vi "GetClassTemplates.vi"(0 "ClassWriterNative in":refnum<class "ClassWriterNative.lvclass">, 1 "DerivedFromThisClass(if any)":refnum<vi>, 5 "error in (no error)":errorcluster) -> (14 "ClassWriterNative out":refnum<class "ClassWriterNative.lvclass">, 15 "Templates":T1[](array[typedef]), 19 "error out":errorcluster)   [LabVIEW 2014, in "ClassWriterNative.lvclass"]
uses:
  <resource>/Framework/Providers/Open_GDS/ClassProviders/Provider_LvNativeClass/ClassWriterNative_class/ClassWriterNative.lvclass
  <resource>/Framework/Providers/Open_GDS/ClassProviders/Provider_BaseClassInterface/ClassTemplateType.ctl
  <resource>/Framework/Providers/Open_GDS/ClassProviders/Common/ScriptingFunctions/Scripting_ConnectorPanePatternType.ctl
  <resource>/Framework/Providers/Open_GDS/ClassProviders/Provider_BaseClassInterface/ClassWriter_class/ClassWriter.lvclass
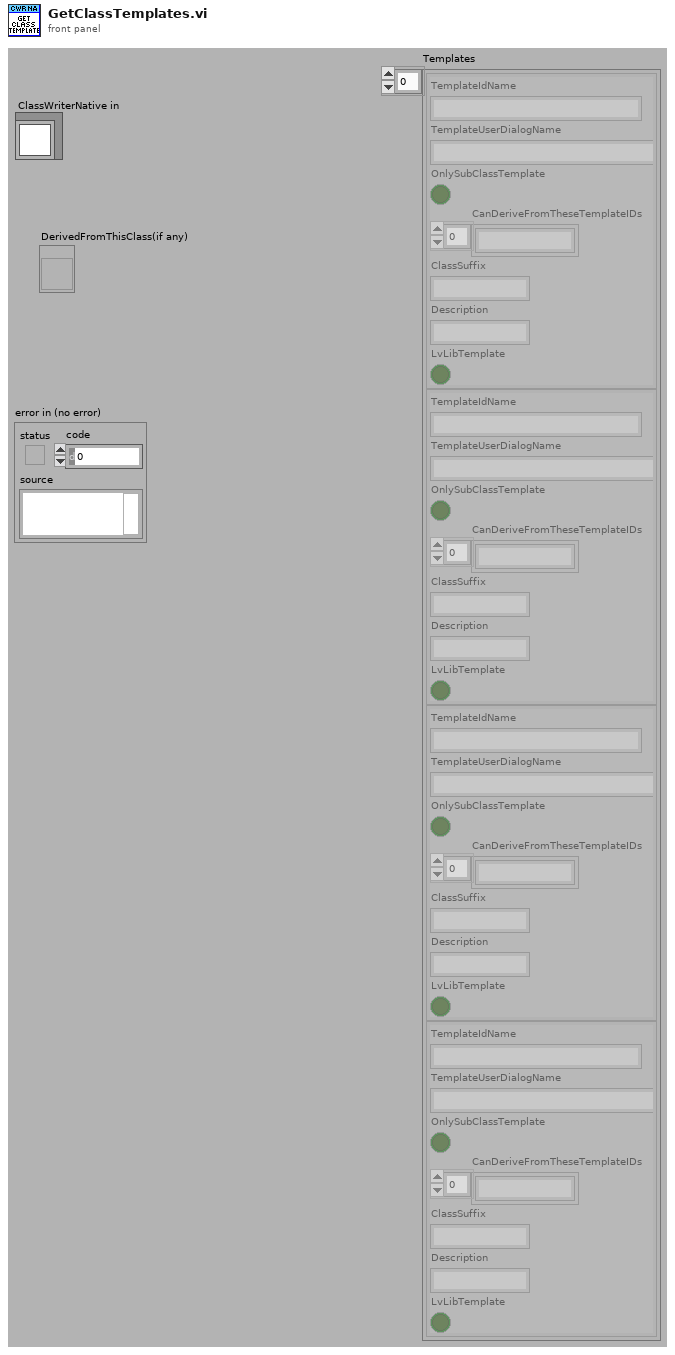
[diagram p1: front panel]
types:
  T1 = typedef "ClassWriter.lvclass/ClassTemplateType.ctl" = cluster{"TemplateIdName":string, "TemplateUserDialogName":string, "OnlySubClassTemplate":bool, "CanDeriveFromTheseTemplateIDs":string[], "ClassSuffix":string, "Description":string, "LvLibTemplate":bool}
  T2 = typedef "Scripting_ConnectorPanePatternType.ctl" = u16
  T3 = typedef "GDSLvCLass_ClassSettingsType.ctl" = cluster{"ClassProviderName":string, "ClassTemplateUsed":string, "ClassTemplateVersion":string, "ClassDescription":string, "PlugIns":T4[], "ConnectorPanePattern":string}
  T4 = typedef "GDSLvClass_PlugIn.ctl" = cluster{"Type":T5, "ID":string, "Version":string, "Path":path, "Name":string, "Data":variant}
  T5 = typedef "GDSLvClass_PlugInTypes.ctl" = enum16{"DesignPattern", "MethodTypes"}
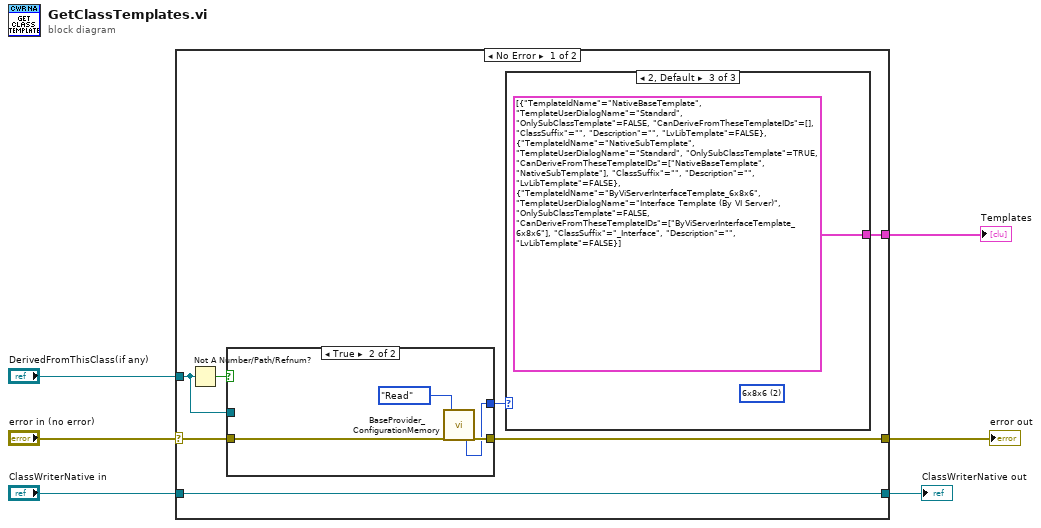
[diagram p0: block diagram]
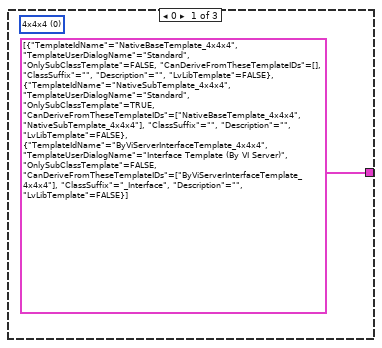
[diagram p2: hidden frame]
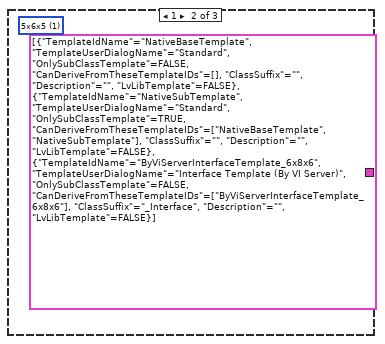
[diagram p3: hidden frame]
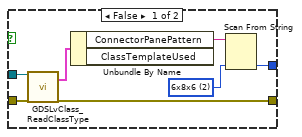
[diagram p4: hidden frame]
diagram:
  n1 = case shown="No Error" "error in (no error)" {
    selector: "error in (no error)" -> [w9 w29]
    tunnel: [w8 w29] -> w5
    tunnel: [w13 w28] -> w3
    tunnel: "ClassWriterNative in" -> [w13 w28]
    tunnel: [w12 _] -> w2
    tunnel: "DerivedFromThisClass(if any)" -> [w10 _]
    frame No Error {
      n2 = Not A Number/Path/Refnum?(number/path/refnum=w10) -> (NaN/Path/Refnum?=w11:bool)
      n3 = case shown="True" w11 {
        tunnel: w9 -> [w20 w26]
        tunnel: w10 -> [w19 _]
        tunnel: [w18 w25] -> w8
        tunnel: [w17 w24] -> w7
        frame False {
          w21 = T2 2 items=["4x4x4", "5x6x5", "6x8x6"] ("Pattern")
          n4 = call <resource>:"GDSLvClass_ReadClassType.vi"("Class Refnum In"=w19, "error in (no error)"=w20) -> ("ClassSettings"=w23:T3, "error out"=w18:errorcluster)  [unwired: 15 in, 1 out]
          n5 = Unbundle By Name(w23) -> ("ConnectorPanePattern"=w22:string)  [unwired: 1 out]
          n6 = Scan From String(input string=w22, default 1=w21) -> (output 1=w17:T2)  [unwired: 3 in, 3 out]
        }
        frame True {
          n7 = call <resource>:"BaseProvider_ConfigurationMemory.vi"("error in (no error)"=w26, "Action"=enum16{"Read", "Load", "Save"}."Read") -> ("PatternOut"=w24:T2, "error out"=w25:errorcluster)  [unwired: 11 in, 5 out]
        }
      }
      n8 = case shown="2, Default" w7 {
        tunnel: [T1[] [{"TemplateIdName"="NativeBaseTemplate_4x4x4", "TemplateUserDialogName"="Standard", "OnlySubClassTemplate"=FALSE, "CanDeriveFromTheseTemplateIDs"=[], "ClassSuffix"="", "Description"="", "LvLibTemplate"=FALSE}, {"TemplateIdName"="NativeSubTemplate_4x4x4", "TemplateUserDialogName"="Standard", "OnlySubClassTemplate"=TRUE, "CanDeriveFromTheseTemplateIDs"=["NativeBaseTemplate_4x4x4", "NativeSubTemplate_4x4x4"], "ClassSuffix"="", "Description"="", "LvLibTemplate"=FALSE}, {"TemplateIdName"="ByViServerInterfaceTemplate_4x4x4", "TemplateUserDialogName"="Interface Template (By VI Server)", "OnlySubClassTemplate"=FALSE, "CanDeriveFromTheseTemplateIDs"=["ByViServerInterfaceTemplate_4x4x4"], "ClassSuffix"="_Interface", "Description"="", "LvLibTemplate"=FALSE}] ("TemplateIdNames") T1[] [{"TemplateIdName"="NativeBaseTemplate", "TemplateUserDialogName"="Standard", "OnlySubClassTemplate"=FALSE, "CanDeriveFromTheseTemplateIDs"=[], "ClassSuffix"="", "Description"="", "LvLibTemplate"=FALSE}, {"TemplateIdName"="NativeSubTemplate", "TemplateUserDialogName"="Standard", "OnlySubClassTemplate"=TRUE, "CanDeriveFromTheseTemplateIDs"=["NativeBaseTemplate", "NativeSubTemplate"], "ClassSuffix"="", "Description"="", "LvLibTemplate"=FALSE}, {"TemplateIdName"="ByViServerInterfaceTemplate_6x8x6", "TemplateUserDialogName"="Interface Template (By VI Server)", "OnlySubClassTemplate"=FALSE, "CanDeriveFromTheseTemplateIDs"=["ByViServerInterfaceTemplate_6x8x6"], "ClassSuffix"="_Interface", "Description"="", "LvLibTemplate"=FALSE}] ("TemplateIdNames") T1[] [{"TemplateIdName"="NativeBaseTemplate", "TemplateUserDialogName"="Standard", "OnlySubClassTemplate"=FALSE, "CanDeriveFromTheseTemplateIDs"=[], "ClassSuffix"="", "Description"="", "LvLibTemplate"=FALSE}, {"TemplateIdName"="NativeSubTemplate", "TemplateUserDialogName"="Standard", "OnlySubClassTemplate"=TRUE, "CanDeriveFromTheseTemplateIDs"=["NativeBaseTemplate", "NativeSubTemplate"], "ClassSuffix"="", "Description"="", "LvLibTemplate"=FALSE}, {"TemplateIdName"="ByViServerInterfaceTemplate_6x8x6", "TemplateUserDialogName"="Interface Template (By VI Server)", "OnlySubClassTemplate"=FALSE, "CanDeriveFromTheseTemplateIDs"=["ByViServerInterfaceTemplate_6x8x6"], "ClassSuffix"="_Interface", "Description"="", "LvLibTemplate"=FALSE}] ("TemplateIdNames")] -> w12
        frame 0 {
          (unwired) T2 0 items=["4x4x4", "5x6x5", "6x8x6"] ("Pattern")
        }
        frame 1 {
          (unwired) T2 1 items=["4x4x4", "5x6x5", "6x8x6"] ("Pattern")
        }
        frame 2, Default {
          (unwired) T2 2 items=["4x4x4", "5x6x5", "6x8x6"] ("Pattern")
        }
      }
    }
    frame Error {
    }
  }
  "error out" <- w5
  "ClassWriterNative out" <- w3
  "Templates" <- w2
